vi "BuildTestFromTheory.vi"(8 "error in (no error)":errorcluster, 10 "VI Refnum":refnum<vi>) -> (0 "error out":errorcluster, 2 "Test":refnum<class "Test.lvclass">)   [LabVIEW 2019, in "LVUnitTestBuilder.lvclass"]
uses:
  LVUnitTestBuilder.lvclass
  Test/Test.lvclass
  Theory/Theory.lvclass
  C:/Users/de200256/Code/neuperger/lvunit/Test/Test.lvclass
  TestSuite/TestSuite.lvclass
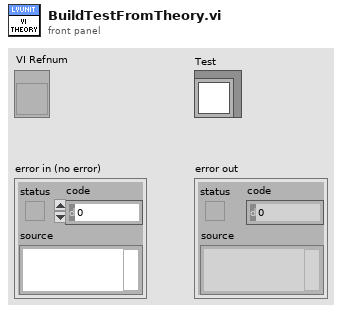
[diagram p1: front panel]
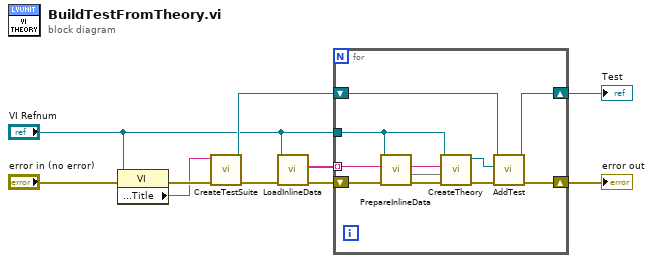
[diagram p0: block diagram]
diagram:
  n1 = property class="VI"(reference="VI Refnum", error in="error in (no error)") -> (error out=w3:errorcluster, "Front Panel.Title"=w1:string)  [unwired: 1 out]
  n2 = call "CreateTestSuite.vi"("error in (no error)"=w3, "Name"=w1) -> ("error out"=w8:errorcluster, "TestSuite"=w7:refnum<class "TestSuite.lvclass">)  [unwired: 8 in]
  n3 = call "LoadInlineData.vi"("error in (no error)"=w8, "VI Refnum"="VI Refnum") -> ("error out"=w10:errorcluster, "Inline Data"=w9:string[])  [unwired: 8 in]
  n4 = for {
    shift-right: [w18] -> w6
    shift-left: w7 -> [w19]
    shift-right: [w20] -> w4
    shift-left: w10 -> [w16]
    tunnel: w9 -> [w14] mode=indexing
    tunnel: "VI Refnum" -> [w11]
    n5 = call "PrepareInlineData.vi"("error in (no error)"=w16, "Inline Data"=w14, "VI Refnum"=w11) -> ("error out"=w15:errorcluster, "Control Data"=w13:map{string, variant}, "Data Name"=w12:string)  [unwired: 6 in]
    n6 = call "CreateTheory.vi"("error in (no error)"=w15, "Control Data"=w13, "Data Name (\"\")"=w12, "VI Refnum"=w11) -> ("error out"=w21:errorcluster, "Theory"=w17:refnum<class "Theory.lvclass">)  [unwired: 6 in]
    n7 = call-dynamic "AddTest.vi"("error in (no error)"=w21, "Test"=w17, "TestSuite in"=w19) -> ("error out"=w20:errorcluster, "TestSuite out"=w18:refnum<class "TestSuite.lvclass">)  [unwired: 7 in]
  }
  "error out" <- w4
  "Test" <- w6
